vi "Test_HMI.vi"() -> ()   [LabVIEW 2016]
panel:
  in  "LC1_reboot":bool
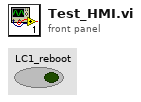
[diagram p1: front panel]
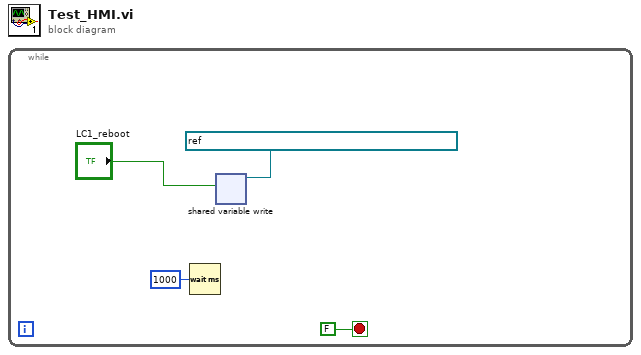
[diagram p0: block diagram]
diagram:
  n1 = while {
    stop <- FALSE stop-if-true
    n2 = Wait (ms)(milliseconds to wait=u32 1000) -> ()  [unwired: 1 out]
    n3 = shared-variable-write(refnum<k21> "ni.var.psp://LC1/Untitled Library 1/LC1_reboot" ("shared variable refnum in"), "LC1_reboot") -> ()  [unwired: 1 in, 2 out]
  }
